vi "PM9_TCP_READ-TEMP.vi"(0 "VISA":refnum<visa-resource-name>="TCPIP0::169.254.70.190::502::SOCKET", 5 "connection ID":refnum<k5>, 11 "error in (no error)":errorcluster, 12 "Sensor":u16(ring)=1 items=["SENSOR 1", "SENSOR 2"], 13 "milliseconds to wait":u32=10, 14 "Close tcp(t)":bool) -> (3 "Value":sgl=25.557514 format="%#.6g", 4 "visa out":refnum<visa-resource-name>="TCPIP0::169.254.70.190::502::SOCKET", 6 "connection ID out":refnum<k5>, 15 "error out":errorcluster)   [LabVIEW 2018]
panel:
  out "resulting string":string
  # "Use a valid connection id to run in loop"
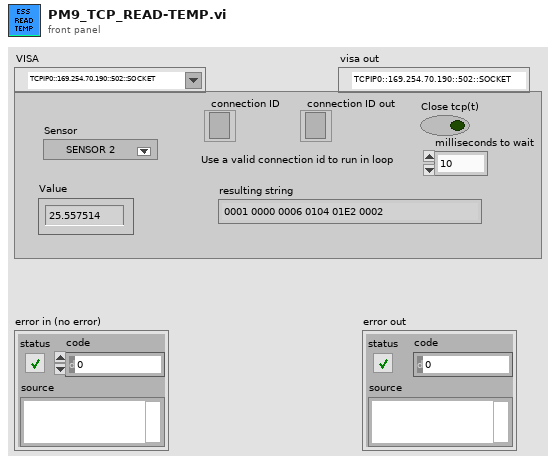
[diagram p1: front panel]
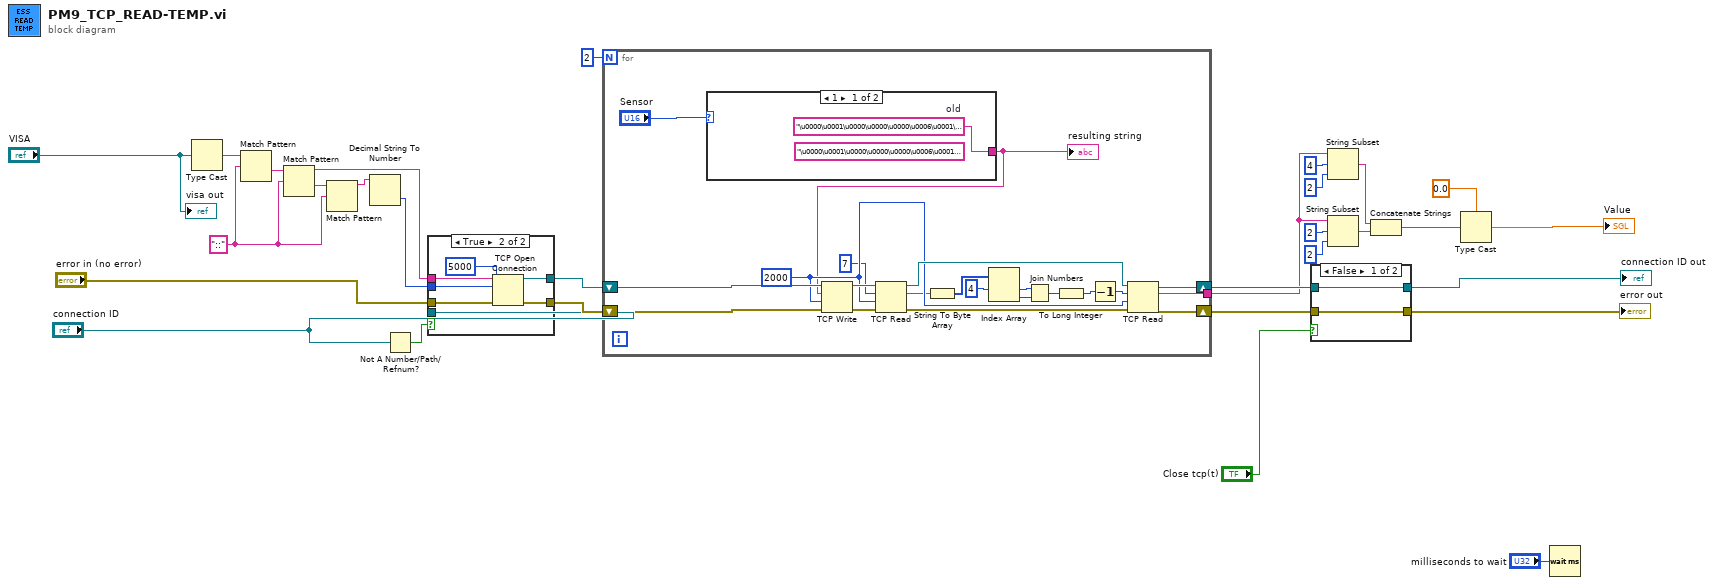
[diagram p0: block diagram]
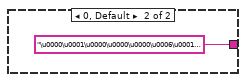
[diagram p2: hidden frame]
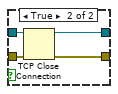
[diagram p4: hidden frame]
diagram:
  w12 = "::" ("search string/char (-)")
  n1 = Type Cast(x="VISA") -> (*(type *) &x=w15:string)  [unwired: 1 in]
  n2 = Match Pattern(string=w15, regular expression=w12) -> (after substring=w14:string)  [unwired: 1 in, 3 out]
  n3 = Match Pattern(string=w14, regular expression=w12) -> (before substring=w10:string, after substring=w13:string)  [unwired: 1 in, 2 out]
  n4 = Match Pattern(string=w13, regular expression=w12) -> (before substring=w11:string)  [unwired: 1 in, 3 out]
  n5 = Decimal String To Number(string=w11) -> (number=w9:i32)  [unwired: 2 in, 1 out]
  n6 = Not A Number/Path/Refnum?(number/path/refnum="connection ID") -> (NaN/Path/Refnum?=w4:bool)
  n7 = case shown="True" w4 {
    tunnel: [w32 w38] -> w30
    tunnel: [w31 w37] -> w29
    tunnel: w10 -> [_ w35]
    tunnel: w9 -> [_ w34]
    tunnel: "error in (no error)" -> [w31 w33]
    tunnel: "connection ID" -> [w32 _]
    frame False {
    }
    frame True {
      n8 = TCP Open Connection(address=w35, remote port or service name=w34, timeout ms (60000)=5000, error in (no error)=w33) -> (connection ID=w38:refnum<k5>, error out=w37:errorcluster)  [unwired: 1 in]
    }
  }
  n9 = for {
    N: 2 -> [_]
    tunnel: [w41] -> w20
    shift-right: [w57] -> w28
    shift-left: w30 -> [w59]
    shift-right: [w56] -> w27
    shift-left: w29 -> [w58]
    w51 = 2000 ("timeout ms (25000)")
    n10 = case shown="1" "Sensor" {
      tunnel: [w60 "\u0000\u0001\u0000\u0000\u0000\u0006\u0001\u0004\u0001h\u0000\u0002" ("address")] -> w40
      frame 1 {
        w60 = "\u0000\u0001\u0000\u0000\u0000\u0006\u0001\u0004\u0001¸\u0000\u0002"  # old
        (unwired) "\u0000\u0001\u0000\u0000\u0000\u0006\u0001\u0004\u0001â\u0000\u0002" ("address")
      }
      frame 0, Default {
      }
    }
    "resulting string" <- w40
    n11 = TCP Write(connection ID=w59, data in=w40, error in (no error)=w58, 9:w51) -> (connection ID out=w55:refnum<k5>, error out=w53:errorcluster)  [unwired: 1 out]
    n12 = TCP Read(connection ID=w55, bytes to read=7, error in (no error)=w53, 9:w51) -> (connection ID out=w54:refnum<k5>, data out=w43:string, error out=w52:errorcluster)  [unwired: 1 in]
    n13 = String To Byte Array(string=w43) -> (unsigned byte array=w44:u8[])
    n14 = Index Array(array=w44, index #1=4 ("index")) -> (element #1=w45:u8, element #2=w46:u8)  [unwired: 1 in]
    n15 = Join Numbers(hi=w45, lo=w46) -> ((hi.lo)=w48:u16)
    n16 = To Long Integer(number=w48) -> (32bit integer=w47:i32)
    n17 = Decrement(x=w47) -> (x-1=w42:i32)
    n18 = TCP Read(connection ID=w54, bytes to read=w42, error in (no error)=w52, 9:w51) -> (connection ID out=w57:refnum<k5>, data out=w41:string, error out=w56:errorcluster)  [unwired: 1 in]
  }
  n19 = case shown="False" "Close tcp(t)" {
    tunnel: w28 -> [w63 w67]
    tunnel: w27 -> [w62 w66]
    tunnel: [w62 w65] -> w2
    tunnel: [w63 w64] -> w7
    frame False {
    }
    frame True {
      n20 = TCP Close Connection(connection ID=w67, error in (no error)=w66) -> (connection ID out=w64:refnum<k5>, error out=w65:errorcluster)  [unwired: 1 in]
    }
  }
  "error out" <- w2
  "connection ID out" <- w7
  n21 = String Subset(string=w20, offset (0)=u16 4 ("bytes to read"), length (rest)=u16 2 ("bytes to read")) -> (substring=w19:string)
  n22 = String Subset(string=w20, offset (0)=u16 2 ("bytes to read"), length (rest)=u16 2 ("bytes to read")) -> (substring=w18:string)
  n23 = Concatenate Strings(w19, w18) -> (w17:string)
  n24 = Type Cast(type=sgl 0.0 ("bytes to read"), x=w17) -> (*(type *) &x=→"Value":sgl)
  n25 = Wait (ms)(milliseconds to wait="milliseconds to wait") -> ()  [unwired: 1 out]
  "visa out" <- "VISA"
